vi "FRC Color Processing Balls Example.vi"() -> ()   [LabVIEW 2019]
uses:
  <vilib>/Rock Robotics/WPI/Camera/WPI_CameraSettings Read MJPG.ctl
  <vilib>/Rock Robotics/WPI/Camera/WPI_CameraImageSize.ctl
  Vision Support Code/Camera Types.ctl
  <vilib>/Rock Robotics/WPI/Camera/WPI_CameraExposure Values.ctl
  <vilib>/Rock Robotics/WPI/Camera/WPI_CameraWhite Balance Values.ctl
  <vilib>/vision/NI_Vision_Development_Module.lvlib
panel:
  out "Disqualified":i32
  in  "Details":bool
  out "Results":T1(array[cluster]) {"Normalized Center"."x" format="%#_2g"; "Normalized Center"."y" format="%#_2g"; "Overall Score" format="%#_2g"; "Distance (ft)" format="%#_3g"; "Area Score" format="%#_2g"; "Moment Score" format="%#_2g"; "Aspect Score" format="%#_2g"}
  in  "Size Limit %":dbl=0.1 min=0.0 max=100.0 step=0.01 format="%#_13g"
  out "Instructions:":string="Instructions:\nUse the Source section to select either a file or camera source. Use files to view a directory of images, or use a built-in, USB, or IP camera on your laptop.\nFiles can be JPEG, BMP, PNG, or AVI movie formats. The camera will be USB 0, USB 1, or an IP.\n\nColor Range can be encoded as HSL or related color modes. HSL is most accurate, but somewhat slower. You can interactively calibrate to the color of the balls or other field elements.\nTo do so, click and draw a line in Original Image to auto-calibrate the color. You may want to widen and tweak Hue, Sat and Val by hand.\nThe Annotate button controls drawing a rectangle and labeling objects with distance and score. Details control the diplay of sub-scores. Distance relies on knowing the Camera Type and lens calibration (it looks up the lens view angle).\n\nThe Size, Count, and Score Limits make the detection more or less picky. Amber color indicates that the limit took effect. Adjust limits as desired.\n\nResults give you the distance to the target, the center in a normalized (-1 to 1) form, scores, and sub-scores.\n\nBe sure to use camera exposure and brightness to help simplify your image and acquire color saturated images.\n\nThere are lots of comments on the diagram to explain the code."
  in  "Color Mode":u16(ring)=2 items=["RGB", "HSL", "HSV", "HSI"]
  in  "Particle Count LImit":i32=5
  in  "Score Threshold %":dbl=75.0
  in  "Std Devs for Calibration":cluster{"H":dbl, "S":dbl, "V":dbl}={"H"=4.0, "S"=8.0, "V"=8.0}
  in  "Camera Type (for distance)":T2=enum."MS HD3000 square"
  in  "Source":enum32{"Files", "Camera"}(tab)
  in  "Play":bool=TRUE
  in  "frame":i32(slide) scale=0.0..851.0
  in  "Images":i32(listbox)
  in  "Folder Location":path=path "C:/Program Files (x86)/National Instruments/LabVIEW 2018/examples/FRC/roboRIO/Vision/2019 Vision Example/Sample Images"
  in  "Camera Settings 1":T3={"fps"=20, "compression"=30, "Image Size"=enum."320x240", "Config Shown"=FALSE}
  in  "Camera Address":string="USB 1"
  in  "Camera Settings 2":T7={"Exposure"=enum."Auto", "Exposure (%)"=50.0, "Brightness"=50, "White Balance"=enum."Auto", "Color Temp (K)"=0.0} {"Brightness" min=0 max=100}
  in  "Annotate":bool=TRUE
  out "Qualified":i32
  in  "Color Range":T8={"Hue"={26.177839279174805, 50.423593521118164}, "Sat"={194.28571428571428, 255.0}, "Val"={69.10978698730469, 253.0}} {"Hue" scale=0.0..255.0 scale format="%#_3g"}
  out "Mask":T9(plugin-control)
  out "Original Image":T9(plugin-control)
  # "Limits"
  # "Particle Results"
  # "Scores"
  # "Good target"
  # "Disqualified"
  # "Distance (ft)"
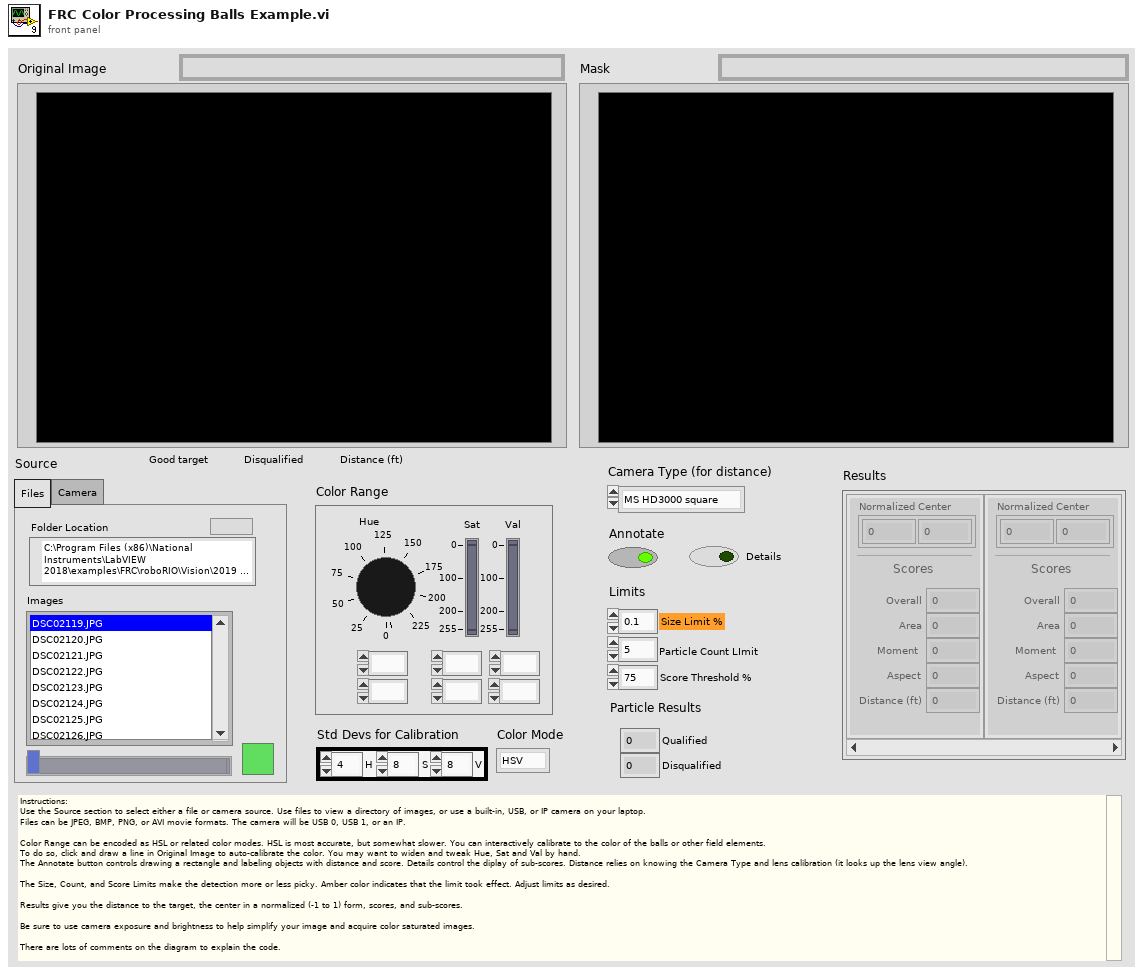
[diagram p1: front panel]
types:
  T1 = cluster{"diameter points":cluster{"first point":cluster{"x":dbl, "y":dbl}, "projected point":cluster{"x":dbl, "y":dbl}}, "Normalized Center":cluster{"x":dbl, "y":dbl}, "Overall Score":dbl, "Area Score":dbl, "Moment Score":dbl, "Aspect Score":dbl, "Distance (ft)":dbl, "Upper Goal":bool}[]
  T2 = typedef "Camera Types.ctl" = enum16{"206", "1011", "1013", "MS HD3000 square", "MS HD3000 640x480"}
  T3 = typedef "WPI_CameraSettings Read MJPG.ctl" = cluster{"fps":i32, "compression":i32, "Image Size":T4, "Config Shown":bool}
  T4 = typedef "WPI_CameraImageSize.ctl" = enum16{"640x480", "320x240", "160x120", "Custom"}
  T5 = typedef "WPI_CameraExposure Values.ctl" = enum16{"Auto", "Flicker-free 50 Hz", "Flicker-free 60 Hz", "Hold current", "Custom"}
  T6 = typedef "WPI_CameraWhite Balance Values.ctl" = enum16{"Auto", "Fixed indoor", "Fixed outdoor 1", "Fixed outdoor 2", "Fixed fluorescent 1", "Fixed fluorescent 2", "Hold current", "Custom"}
  T7 = cluster{"Exposure":T5, "Exposure (%)":dbl, "Brightness":i32, "White Balance":T6, "Color Temp (K)":dbl}
  T8 = cluster{"Hue":cluster{dbl, dbl}, "Sat":cluster{dbl, dbl}, "Val":cluster{dbl, dbl}}
  T9 = typedef "IMAQ Image.ctl" = refnum<image>
  T10 = typedef "Particle Parameters" = i32
  T11 = typedef "Image Type" = u32
  T12 = enum8{"Enabled", "Disabled", "Disabled and Grayed Out"}
  T13 = cluster{cluster{dbl, dbl}, cluster{dbl, dbl}, cluster{dbl, dbl}}
  T14 = cluster{"remainder":i32, "size":bool, "count":bool}
  T15 = typedef "Target Fields.ctl" = cluster{"diameter points":cluster{"first point":cluster{"x":dbl, "y":dbl}, "projected point":cluster{"x":dbl, "y":dbl}}, "normalized center":cluster{"x":dbl, "y":dbl}, "Overall Score":dbl, "Area Score":dbl, "Moment Score":dbl, "Aspect Score":dbl, "Distance (ft)":dbl, "Upper Goal":bool}
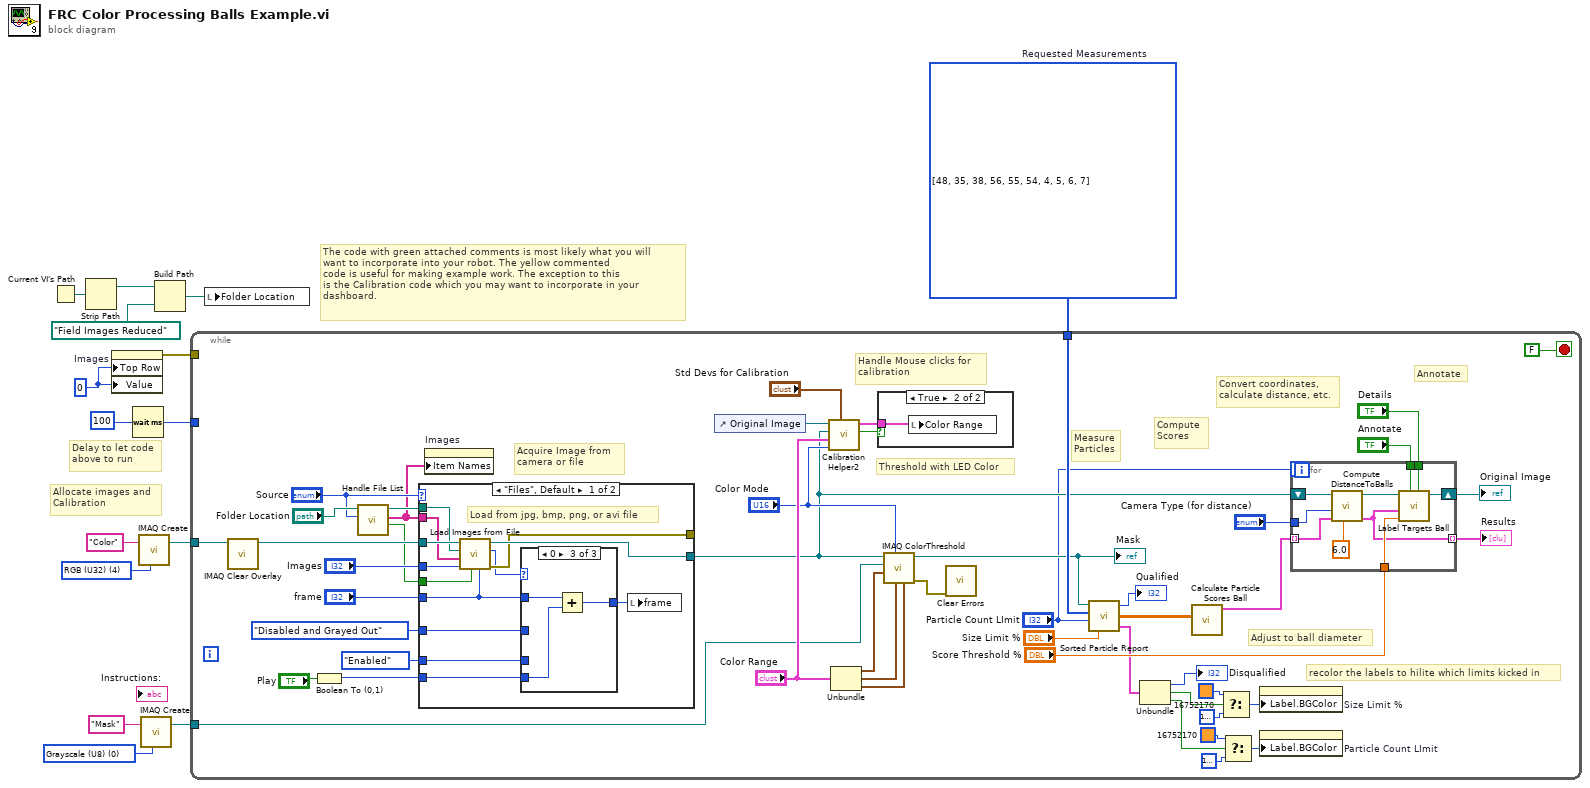
[diagram p0: block diagram]
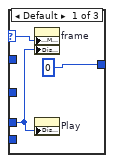
[diagram p2: hidden frame]
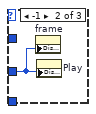
[diagram p3: hidden frame]
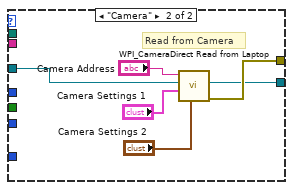
[diagram p4: hidden frame]
diagram:
  w6 = u32 0 ("milliseconds to wait")
  w10 = T10[] [48, 35, 38, 56, 55, 54, 4, 5, 6, 7] items=["Center of Mass X", "Center of Mass Y", "First Pixel X", "First Pixel Y", "Bounding Rect Left", "Bounding Rect Top", "Bounding Rect Right", "Bounding Rect Bottom", "Max Feret Diameter Start X", "Max Feret Diameter Start Y", "Max Feret Diameter End X", "Max Feret Diameter End Y", "Max Horiz. Segment Length Left", "Max Horiz. Segment Length Right", "Max Horiz. Segment Length Row", "-", "Bounding Rect Width", "Bounding Rect Height", "Bounding Rect Diagonal", "Perimeter", "Convex Hull Perimeter", "Holes' Perimeter", "Max Feret Diameter", "Equivalent Ellipse Major Axis", "Equivalent Ellipse Minor Axis", "Equivalent Ellipse Minor Axis (Feret)", "Equivalent Rect Long Side", "Equivalent Rect Short Side", "Equivalent Rect Diagonal", "Equivalent Rect Short Side (Feret)", "Average Horiz. Segment Length", "Average Vert. Segment Length", "Hydraulic Radius", "Waddel Disk Diameter", "-", "Area", "Holes' Area", "Particle & Holes' Area", "Convex Hull Area", "Image Area", "-", "Number of Holes", "Number of Horiz. Segments", "Number of Vert. Segments", "-", "Orientation", "Max Feret Diameter Orientation", "-", "% Area/Image Area", "% Area/(Particle & Holes' Area)", "Ratio of Equivalent Ellipse Axes", "Ratio of Equivalent Rect Sides", "-", "Elongation Factor", "Compactness Factor", "Heywood Circularity Factor", "Type Factor", "-", "Sum X", "Sum Y", "Sum XX", "Sum XY", "Sum YY", "Sum XXX", "Sum XXY", "Sum XYY", "Sum YYY", "-", "Moment of Inertia XX", "Moment of Inertia XY", "Moment of Inertia YY", "Moment of Inertia XXX", "Moment of Inertia XXY", "Moment of Inertia XYY", "Moment of Inertia YYY", "Norm. Moment of Inertia XX", "Norm. Moment of Inertia XY", "Norm. Moment of Inertia YY", "Norm. Moment of Inertia XXX", "Norm. Moment of Inertia XXY", "Norm. Moment of Inertia XYY", "Norm. Moment of Inertia YYY", "Hu Moment 1", "Hu Moment 2", "Hu Moment 3", "Hu Moment 4", "Hu Moment 5", "Hu Moment 6", "Hu Moment 7"]  # Requested Measurements
  w13 = T11 0 items=["Grayscale (U8)", "Grayscale (I16)", "Grayscale (SGL)", "Complex (CSG)", "RGB (U32)", "HSL (U32)", "RGB (U64)", "Grayscale (U16)"] ("Image Type")
  w14 = T11 4 items=["Grayscale (U8)", "Grayscale (I16)", "Grayscale (SGL)", "Complex (CSG)", "RGB (U32)", "HSL (U32)", "RGB (U64)", "Grayscale (U16)"] ("Image Type")
  # "Delay to let code\nabove to run"
  # "The code with green attached comments is most likely what you will\nwant to incorporate into your robot. The yellow commented\ncode is useful for making example work. The exception to this\nis the Calibration code which you may want to incorporate in your\ndashboard."
  # "Allocate images and\nCalibration"
  n1 = Current VI's Path() -> (path=w9:path)
  n2 = Strip Path(path=w9) -> (stripped path=w7:path)  [unwired: 1 out]
  n3 = property on="Images" class="LstBox (strict)"("Top Row"=w6, "Value"=w6) -> (error out=w1:errorcluster)  [unwired: 2 in, 1 out]
  n4 = Wait (ms)(milliseconds to wait=u32 100) -> (millisecond timer value=w3:u32)
  n5 = call "IMAQ Create"("Image Name"="Color", "Image Type"=w14) -> ("New Image"=w5:T9)  [unwired: 2 in, 2 out]
  n6 = call "IMAQ Create"("Image Name"="Mask", "Image Type"=w13) -> ("New Image"=w11:T9)  [unwired: 2 in, 2 out]
  n7 = Build Path(base path=w7, name or relative path=path "Field Images Reduced" ("Folder Location")) -> (appended path=w4:path)
  n8 = while {
    tunnel: w5 -> [w46]
    tunnel: w11 -> [w32]
    tunnel: w10 -> [w59]
    tunnel: w3 -> [_]
    tunnel: w1 -> [_]
    stop <- FALSE stop-if-true
    # "recolor the labels to hilite which limits kicked in"
    # "Adjust to ball diameter"
    # "Handle Mouse clicks for\ncalibration"
    # "Measure\nParticles"
    # "Convert coordinates,\ncalculate distance, etc."
    # "Annotate"
    # "Compute\nScores"
    # "Threshold with LED Color"
    # "Acquire Image from\ncamera or file"
    n9 = call "IMAQ Clear Overlay"("Image"=w46) -> ("Image Out"=w45:T9)  [unwired: 2 in, 8 out]
    n10 = Boolean To (0,1)(Boolean="Play") -> (0, 1=w33:i16)
    n11 = call "Handle File List.vi"("Source"="Source", "Folder Location in"="Folder Location") -> ("force"=w28:bool, "filenames"=w29:string[], "Folder Location out"=w38:path)  [unwired: 7 in]
    n12 = case shown="\"Files\", Default" "Source" {
      tunnel: [w76 w90] -> _
      tunnel: [w77 w89] -> w47
      tunnel: w45 -> [w75 w88]
      tunnel: w29 -> [w72 _]
      tunnel: "Images" -> [w74 _]
      tunnel: w38 -> [w73 _]
      tunnel: "frame" -> [w69 _]
      tunnel: w33 -> [w68 _]
      tunnel: T12."Disabled and Grayed Out" ("Disabled") -> [w67 _]
      tunnel: T12."Enabled" ("Disabled") -> [w66 _]
      tunnel: w28 -> [w65 _]
      frame "Files", Default {
        # "Load from jpg, bmp, png, or avi file"
        n13 = call "Load Images from File.vi"("frame"=w69, "Force Load"=w65, "Images"=w74, "image files"=w72, "Folder Location"=w73, "Refnum in"=w75) -> ("error out"=w76:errorcluster, "Number of Frames"=w71:i32, "Refnum out"=w77:T9)  [unwired: 3 in]
        n14 = case shown="0" w71 {
          selector: w71 -> [w80 _ _]
          tunnel: [0 _ w82] -> w70
          tunnel: w69 -> [_ _ w84]
          tunnel: w68 -> [_ _ w83]
          tunnel: w66 -> [w78 _ _]
          tunnel: w67 -> [_ w81 _]
          frame Default {
            n15 = property on="frame" class="Slide (strict)"("Scale.Maximum"=w80, "DisabledEnum"=w78) -> ()  [unwired: 2 in, 2 out]
            n16 = property on="Play" class="Bool (strict)"("DisabledEnum"=w78) -> ()  [unwired: 2 in, 2 out]
          }
          frame -1 {
            n17 = property on="frame" class="Slide (strict)"("DisabledEnum"=w81) -> ()  [unwired: 2 in, 2 out]
            n18 = property on="Play" class="Bool (strict)"("DisabledEnum"=w81) -> ()  [unwired: 2 in, 2 out]
          }
          frame 0 {
            n19 = Add(x=w84, y=w83) -> (x+y=w82:i32)
          }
        }
        n20 = local write "frame"(w70) -> ()
      }
      frame "Camera" {
        # "Read from Camera"
        n21 = call <vilib>:"WPI_CameraDirect Read from Laptop.vi"("Camera Settings 2"="Camera Settings 2", "Camera Settings"="Camera Settings 1", "Image"=w88, "address"="Camera Address") -> ("error out"=w90:errorcluster, "Image Out"=w89:T9)  [unwired: 6 in]
      }
    }
    n22 = property on="Images" class="LstBox (strict)"("Item Names"=w29) -> ()  [unwired: 2 in, 2 out]
    n23 = control-ref of="Original Image"() -> (w56:refnum<vi>)
    n24 = call "Calibration Helper2.vi"("Std Devs"="Std Devs for Calibration", "Color Mode"="Color Mode", "Color Components"="Color Range", "Image"=w47, "Image Ctl Refnum"=w56) -> ("Changed"=w55:bool, "output color"=w54:T13)  [unwired: 5 in]
    n25 = Unbundle("Color Range") -> ("Hue"=w62:cluster{dbl, dbl}, "Sat"=w61:cluster{dbl, dbl}, "Val"=w60:cluster{dbl, dbl})
    n26 = case shown="True" w55 {
      tunnel: w54 -> [_ w91]
      frame False {
      }
      frame True {
        n27 = local write "Color Range"(w91) -> ()
      }
    }
    n28 = call "IMAQ ColorThreshold"("Blue or Luma or Val or Inten Range"=w60, "Green or Sat Range"=w61, "Color Mode"="Color Mode", "Red or Hue Range"=w62, "Image Dst"=w32, "Image Src"=w47) -> ("error out"=w41:errorcluster, "Image Dst Out"=w42:T9)  [unwired: 4 in]
    "Mask" <- w42
    n29 = call <vilib>:"Clear Errors.vi"("error in (no error)"=w41) -> ()  [unwired: 5 in, 2 out]
    n30 = call "Sorted Particle Report.vi"("Min Area Size %"="Size Limit %", "Particle Count Limit"="Particle Count LImit", "Pixel Measurements"=w59, "Image in"=w42) -> ("limits"=w26:T14, "Sorted Data"=w40:dbl[][], "Particles"=→"Qualified":i32)
    n31 = Unbundle(w26) -> ("remainder"=→"Disqualified":i32, "size"=w21:bool, "count"=w18:bool)
    n32 = call "Calculate Particle Scores Ball.vi"("Sorted Data"=w40) -> ("Scores"=w39:T15[])  [unwired: 10 in]
    n33 = Select(t=u32 16752170 ("Color"), s=w21, f=u32 16777216 ("Color")) -> (s? t:f=w20:u32)
    n34 = Select(t=u32 16752170 ("Color"), s=w18, f=u32 16777216 ("Color")) -> (s? t:f=w17:u32)
    n35 = property on="Size Limit %" class="DigNum (strict)"("Label.BGColor"=w20) -> ()  [unwired: 2 in, 2 out]
    n36 = property on="Particle Count LImit" class="DigNum (strict)"("Label.BGColor"=w17) -> ()  [unwired: 2 in, 2 out]
    n37 = for {
      N: "Particle Count LImit" -> [_]
      tunnel: w39 -> [w99] mode=indexing
      tunnel: "Camera Type (for distance)" -> [w96]
      tunnel: "Annotate" -> [w93]
      shift-right: [w101] -> w48
      shift-left: w47 -> [w95]
      tunnel: "Score Threshold %" -> [w100]
      tunnel: [w98] -> w43 mode=indexing
      tunnel: "Details" -> [w92]
      n38 = call "Compute DistanceToBalls.vi"("Target Width (in)"=6.0, "results"=w99, "Camera Type"=w96, "Image Src"=w95) -> ("results out"=w98:T15, "Image Dst Out"=w97:T9)  [unwired: 6 in]
      n39 = call "Label Targets Ball.vi"("Details"=w92, "Annotate"=w93, "Score Threshold"=w100, "results"=w98, "Image in"=w97) -> ("Image out"=w101:T9)  [unwired: 6 in]
    }
    "Original Image" <- w48
    "Results" <- w43
  }
  n40 = local write "Folder Location"(w4) -> ()
